vi "MUX Button Colors.vi"(10 "Color":u32(colorbox)) -> (2 "MUX Button Colors":cluster{"Shadow":u32, "Shadow":u32}[](array[cluster]))   [LabVIEW 2022 SP3, in "TouchControl.lvlib"]
uses:
  TouchControl.lvlib
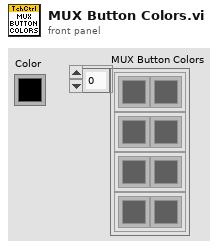
[diagram p1: front panel]
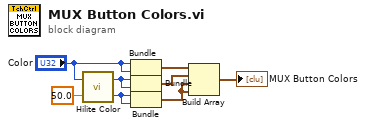
[diagram p0: block diagram]
diagram:
  n1 = call <vilib>:"Hilite Color.vi"("Percentage(30)"=50.0, "Color In"="Color") -> ("Shadow"=w7:u32, "Hilite"=w8:u32)
  n2 = Bundle("Color"="Color", "Color"="Color") -> (w5:cluster{"Color":u32, "Color":u32})  [unwired: 1 in]
  n3 = Bundle("Hilite"=w8, "Hilite"=w8) -> (w4:cluster{"Hilite":u32, "Hilite":u32})  [unwired: 1 in]
  n4 = Bundle("Shadow"=w7, "Shadow"=w7) -> (w3:cluster{"Shadow":u32, "Shadow":u32})  [unwired: 1 in]
  n5 = Build Array(w5, w4, w3, w3) -> (→"MUX Button Colors":cluster{"Shadow":u32, "Shadow":u32}[])
